vi "Find_monitor_from_point.vi"(11 "Point":cluster{"Left":i16, "Top":i16}) -> (2 "In Monitor":bool, 3 "Monitor":i32)   [LabVIEW 2015]
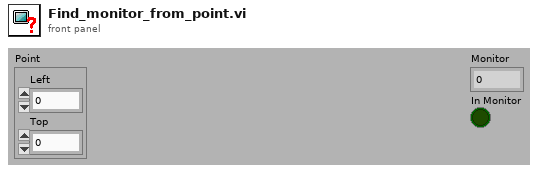
[diagram p1: front panel]
types:
  T1 = typedef "LVAllMonitorsDisplayTypeDef.ctl" = cluster{"Bounds":cluster{"Left":i16, "Top":i16, "Right":i16, "Bottom":i16}, "Depth":i16}[]
  T2 = cluster{"Left":i16, "Top":i16, "Right":i16, "Bottom":i16}
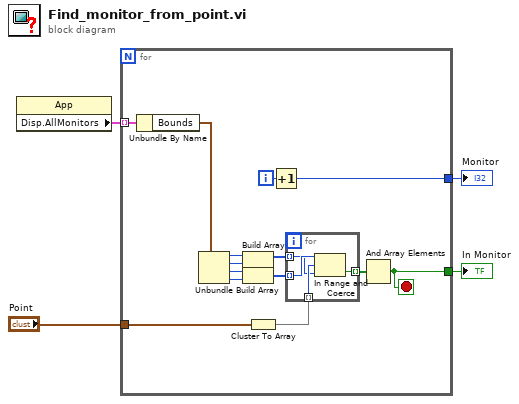
[diagram p0: block diagram]
diagram:
  n1 = property class="App"() -> ("Disp.AllMonitors"=w4:T1)  [unwired: 2 in, 2 out]
  n2 = for {
    tunnel: w4 -> [w18] mode=indexing
    tunnel: [w11] -> w2
    tunnel: "Point" -> [w10]
    tunnel: [w5] -> w1
    i -> [w12]
    stop <- w5 stop-if-true
    n3 = Unbundle By Name(w18) -> ("Bounds"=w13:T2)
    n4 = Unbundle(w13) -> ("Left"=w17:i16, "Top"=w16:i16, "Right"=w15:i16, "Bottom"=w14:i16)
    n5 = Build Array(w17, w16) -> (w9:i16[])
    n6 = Build Array(w15, w14) -> (w8:i16[])
    n7 = Cluster To Array(cluster=w10) -> (array=w7:i16[])
    n8 = Increment(x=w12) -> (x+1=w11:i32)
    n9 = for {
      tunnel: w9 -> [w19] mode=indexing
      tunnel: w8 -> [w20] mode=indexing
      tunnel: w7 -> [w22] mode=indexing
      tunnel: [w21] -> w6 mode=indexing
      n10 = In Range and Coerce(upper limit=w20, x=w22, lower limit=w19) -> (In Range?=w21:bool)  [unwired: 1 out]
    }
    n11 = And Array Elements(Boolean array=w6) -> (logical AND=w5:bool)
  }
  "Monitor" <- w2
  "In Monitor" <- w1
